vi "twoBytesToU16.vi"(2 "LSB":u8, 3 "MSB":u8) -> (1 "Word":u16)   [LabVIEW 2014]
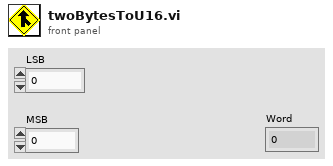
[diagram p1: front panel]
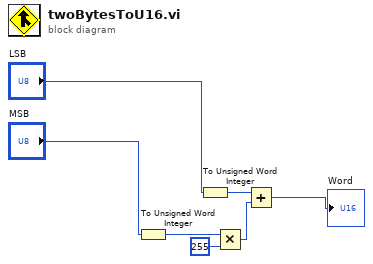
[diagram p0: block diagram]
diagram:
  n1 = To Unsigned Word Integer(number="MSB") -> (unsigned 16bit integer=w7:u16)
  n2 = To Unsigned Word Integer(number="LSB") -> (unsigned 16bit integer=w5:u16)
  n3 = Multiply(x=w7, y=u8 255) -> (x*y=w6:u16)
  n4 = Add(x=w5, y=w6) -> (x+y=→"Word":u16)
